vi "Activate Menu.vi"(8 "error in (no error)":errorcluster, 9 "Run Mode?":bool, 10 "MenuRef":refnum<k9>, 11 "2D Compass.lvclass in":refnum<class "2D Compass.lvclass">) -> (0 "error out":errorcluster, 3 "2D Compass.lvclass out":refnum<class "2D Compass.lvclass">)   [LabVIEW 2017, in "2D Compass.lvclass"]
uses:
  <vilib>/Math Plots/2D Math Plots/2D Compass/2D Compass/2D Compass.lvclass
  e:/builds/penguin/labview/branches/2017/dev/dist/vi.lib/Math Plots/2D Math Plots/2D Plot/2D Plot/2D Plot.lvclass
  <vilib>/Math Plots/2D Math Plots/2D Compass/2D Compass/2D Compass.lvclass/2D Compass.ctl
  <vilib>/Math Plots/2D Math Plots/2D Plot/2D Plot/2D Plot.lvclass
panel:
  in  "New Item Names":string="Auto Size Plot Legend"
  in  "Run-time Menu":T1(array[cluster])=[{"menu tag"="", "items to delete"=["APP_SC_CLEAR_GRAPH", "APP_SC_AUTOSCALE_X", "APP_SC_AUTOSCALE_Y", "APP_SC_SMOOTH_UPDATES", "APP_SC_OPTIONAL_PLANE", "APP_SC_SHOW_DIAGRAM"], "new menu"=[{"item names"="Clear Graph", "item tags"="USER_SC_CLEAR_GRAPH", "after item"="APP_SC_CLEAR_GRAPH"}, {"item names"="Autoscale Magnitude", "item tags"="USER_SC_AUTOSCALE", "after item"="APP_SEPERATOR"}], "root?"=TRUE}, {"menu tag"="APP_SC_VISIBLE_ITEMS", "items to delete"=["APP_SC_PLOT_LEGEND", "APP_SC_SCALE_LEGEND", "APP_SC_GRAPH_PALETTE", "APP_SC_CURSOR_LEGEND", "APP_SC_X_SCROLLBAR", "APP_SC_X_SCALE", "APP_SC_Y_SCALE", "APP_SC_UNIT_LABEL"], "new menu"=[{"item names"="Plot Legend", "item tags"="USER_SC_PLOT_LEGEND", "after item"="APP_SC_SEPERATOR"}, {"item names"="Scale Legend", "item tags"="USER_SC_SCALE_LEGEND", "after item"="USER_SC_PLOT_LEGEND"}, {"item names"="Graph Palette", "item tags"="USER_SC_GRAPH_PALETTE", "after item"="USER_SC_SCALE_LEGEND"}, {"item names"="Cursor Legend", "item tags"="USER_SC_CURSOR_LEGEND", "after item"="USER_SC_GRAPH_PALETTE"}, {"item names"="X Scrollbar", "item tags"="USER_SC_X_SCROLLBAR", "after item"="USER_SC_CURSOR_LEGEND"}, {"item names"="-", "item tags"="APP_SC_SEPERATOR", "after item"="USER_SC_X_SCROLLBAR"}, {"item names"="Magnitude Scale", "item tags"="USER_SC_MAGNITUDE_SCALE", "after item"="APP_SC_SEPERATOR"}, {"item names"="Phase Scale", "item tags"="USER_SC_PHASE_SCALE", "after item"="USER_SC_MAGNITUDE_SCALE"}], "root?"=FALSE}]
  in  "Edit-time Menu":T1(array[cluster])=[{"menu tag"="", "items to delete"=["APP_SC_AUTOSCALE_X", "APP_SC_AUTOSCALE_Y", "APP_SC_SMOOTH_UPDATES", "APP_SC_OPTIONAL_PLANE", "APP_SC_PROPERTIES"], "new menu"=[{"item names"="Autoscale Magnitude", "item tags"="USER_SC_AUTOSCALE", "after item"="APP_SC_AUTOSCALE_X"}, {"item names"="Properties", "item tags"="USER_SC_PROPERTIES", "after item"="APP_SC_SEPARATOR"}], "root?"=TRUE}, {"menu tag"="APP_SC_VISIBLE_ITEMS", "items to delete"=["APP_SC_PLOT_LEGEND", "APP_SC_SCALE_LEGEND", "APP_SC_GRAPH_PALETTE", "APP_SC_CURSOR_LEGEND", "APP_SC_X_SCROLLBAR", "APP_SC_X_SCALE", "APP_SC_Y_SCALE", "APP_SC_UNIT_LABEL"], "new menu"=[{"item names"="Plot Legend", "item tags"="USER_SC_PLOT_LEGEND", "after item"="APP_SC_SEPERATOR"}, {"item names"="Scale Legend", "item tags"="USER_SC_SCALE_LEGEND", "after item"="USER_SC_PLOT_LEGEND"}, {"item names"="Graph Palette", "item tags"="USER_SC_GRAPH_PALETTE", "after item"="USER_SC_SCALE_LEGEND"}, {"item names"="Cursor Legend", "item tags"="USER_SC_CURSOR_LEGEND", "after item"="USER_SC_GRAPH_PALETTE"}, {"item names"="X Scrollbar", "item tags"="USER_SC_X_SCROLLBAR", "after item"="USER_SC_CURSOR_LEGEND"}, {"item names"="-", "item tags"="APP_SC_SEPERATOR", "after item"="USER_SC_X_SCROLLBAR"}, {"item names"="Magnitude Scale", "item tags"="USER_SC_MAGNITUDE_SCALE", "after item"="APP_SC_SEPERATOR"}, {"item names"="Phase Scale", "item tags"="USER_SC_PHASE_SCALE", "after item"="USER_SC_MAGNITUDE_SCALE"}], "root?"=FALSE}, {"menu tag"="APP_SC_ADVANCED", "items to delete"=["APP_SC_SHOW_DIAGRAM"], "new menu"=[], "root?"=FALSE}]
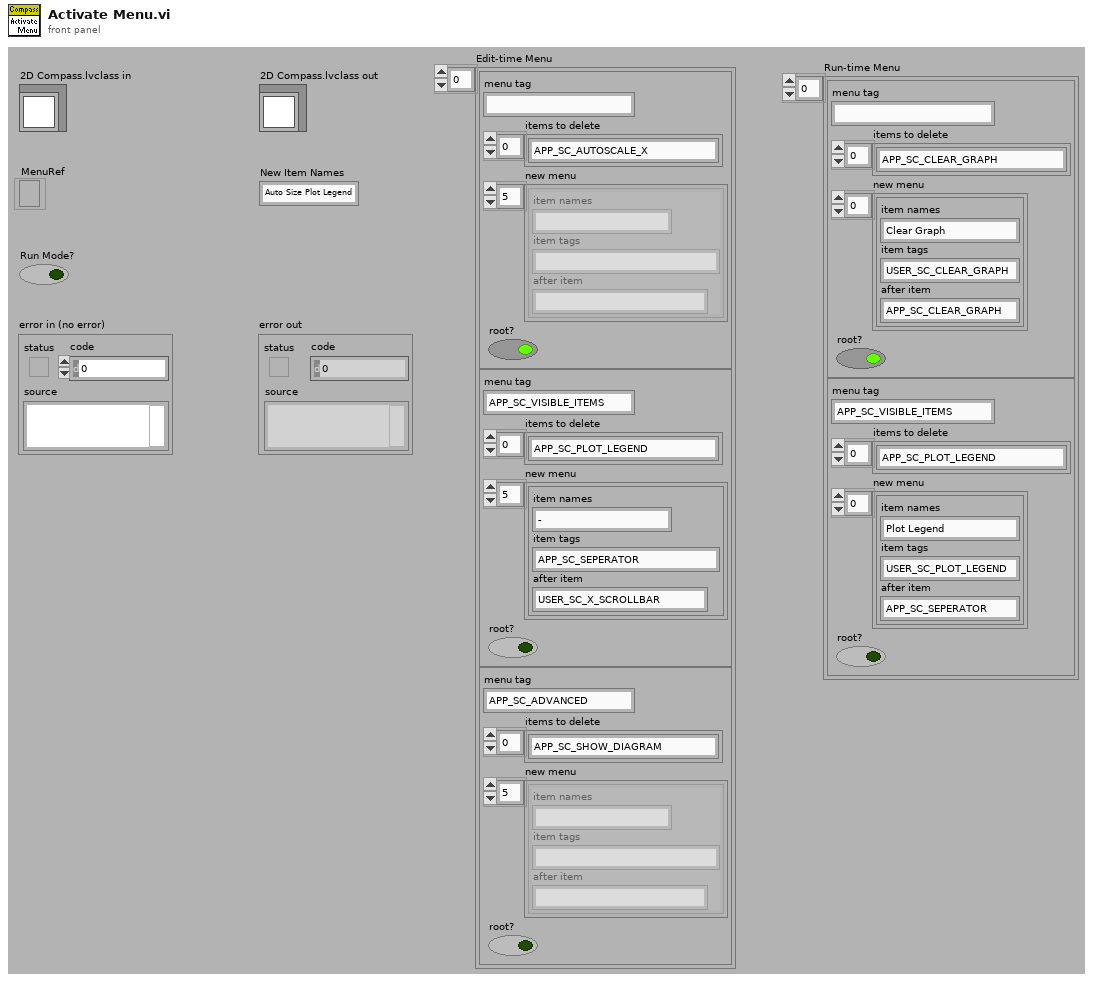
[diagram p1: front panel]
types:
  T1 = cluster{"menu tag":string, "items to delete":string[], "new menu":cluster{"item names":string, "item tags":string, "after item":string}[], "root?":bool}[]
  T2 = typedef "2D Plot.lvclass/Property Cluster.ctl" = cluster{"Graph General":T3, "Format Property":string[], "Scale Array":T4, "Cursor Property":T7, "Annotation List":T9, "Active Cursor":i32, "Active Plot":i32}
  T3 = typedef "2D Plot.lvclass/Graph General Property.ctl" = cluster{"Palette Visible":cluster{"Graph Legend":bool, "Plot Legend":bool, "Auto size":bool, "Number of Plots":u32, "X Scrollbar":bool, "Scale Legend":bool, "Cursor Legend":bool}, "Plot Area Color":cluster{"FG Color":u32, "BG Color":u32}, "Bounds Size":cluster{"Width":u32, "Height":u32}, "Plot Area Bounds":cluster{"Left":i16, "Top":i16, "Right":i16, "Bottom":i16}}
  T4 = typedef "2D Plot.lvclass/Scale Array.ctl" = T5[]
  T5 = typedef "2D Plot.lvclass/Scale Cluster.ctl" = cluster{"General":cluster{"Editable":bool, "Flipped":bool, "Mapping Mode":u8, "Visible":bool, "Style":u8, "Scale Fit":u8}, "Offset and Multiplier":T6, "Range":cluster{"Minimum":dbl, "Maximum":dbl, "Increment":dbl, "Minor Increment":dbl, "Start":dbl}, "Tick Color":cluster{"Major Color":u32, "Minor Color":u32}, "Gird Color":cluster{"Major Color":u32, "Minor Color":u32}, "Marker":cluster{"Visible":bool, "FG Color":u32, "BG Color":u32, "Font Name":string, "Font Size":u32, "Font Bold":bool, "Font Italic":bool, "Font Strikeout":bool, "Font Underline":bool}, "Name Label":cluster{"Visible":bool, "FG Color":u32, "BG Color":u32, "Font Name":string, "Font Size":u32, "Font Bold":bool, "Font Italic":bool, "Font Strikeout":bool, "Font Underline":bool, "Justification":enum16{"Left", "Center", "Right"}, "Text":string}}
  T6 = typedef "LVOffsetAndMultiplierTypeDef.ctl" = cluster{"Offset":dbl, "Multiplier":dbl}
  T7 = typedef "2D Plot.lvclass/Cursor Property.ctl" = cluster{"Cursor List":T8, "Cursor List Addtional":cluster{"Cursor Selection Color":u32, "Line Style":u8, "Line Width":u8, "Visible":bool}[]}
  T8 = typedef "LVCursorListTypeDef.ctl" = cluster{"Name":string, "Color":u32, "Style":u8, "Point Style":u8, "Name Visible":bool, "Allow Drag":bool, "Cursor Mode":u32, "Plot":i32, "Index":i32, "Position":cluster{"X":dbl, "Y":dbl}, "X Scale":u32, "Y Scale":u32, "Watch Plots":i32[], "Watch All Plots":bool, "Plot Area":i32, "Label Offset":cluster{"X":dbl, "Y":dbl}}[]
  T9 = typedef "LVAnnotationListTypeDef.ctl" = cluster{"Name":string, "Color":u32, "Style":u8, "Point Style":u8, "Name Visible":bool, "Allow Drag":bool, "Annotation Mode":u32, "Plot":i32, "Index":i32, "Position":cluster{"X":dbl, "Y":dbl}, "X Scale":u32, "Y Scale":u32, "Show Arrow":bool, "Lock Name":bool, "Plot Area":i32, "Label Offset":cluster{"X":dbl, "Y":dbl}}[]
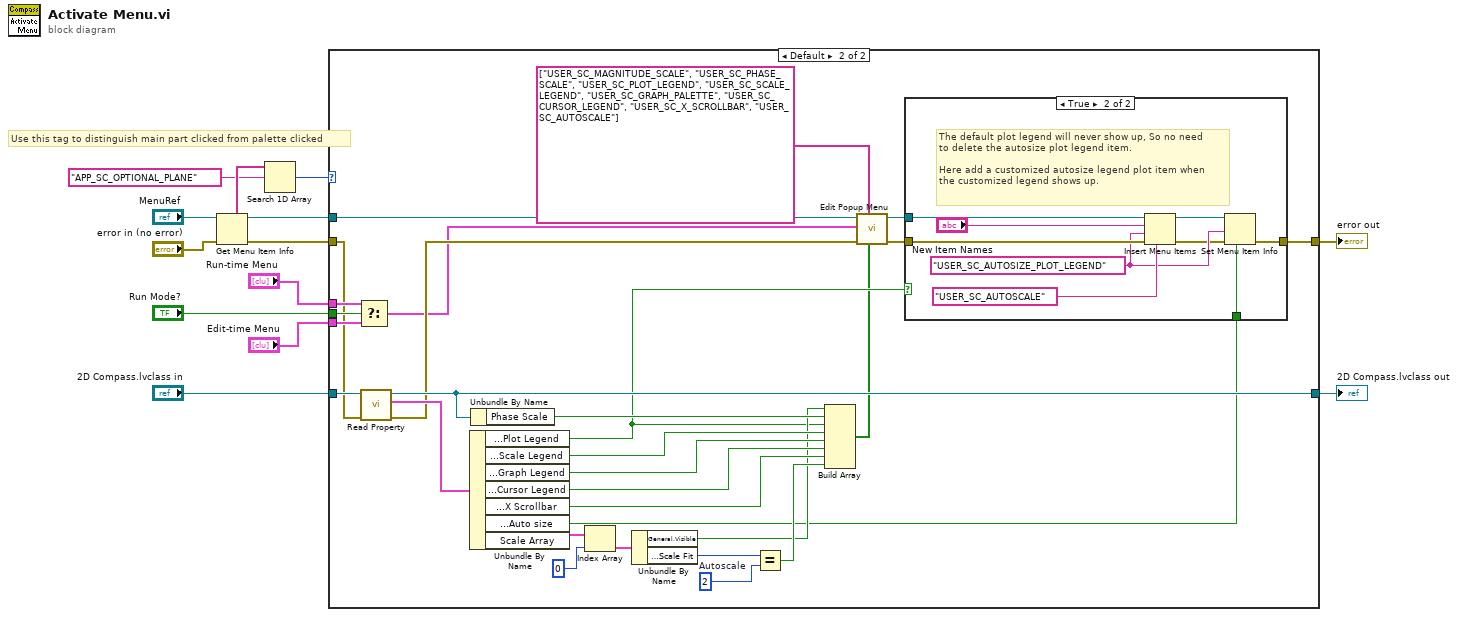
[diagram p0: block diagram]
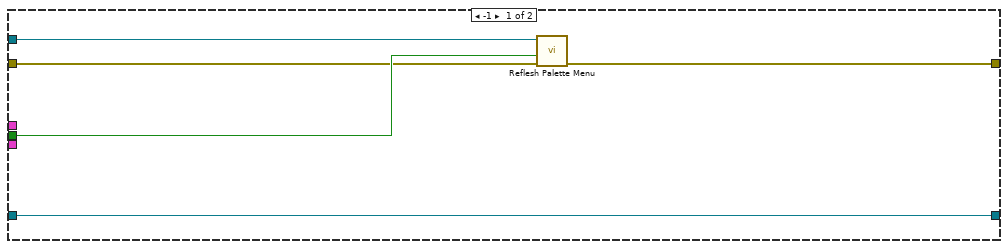
[diagram p2: hidden frame]
diagram:
  # "Use this tag to distinguish main part clicked from palette clicked"
  n1 = Get Menu Item Info(8:"error in (no error)", 11:"MenuRef") -> (0:w1:errorcluster, 3:w6:refnum<k9>, 5:w5:string[])  [unwired: 5 out]
  n2 = Search 1D Array(1D array=w5, element="APP_SC_OPTIONAL_PLANE") -> (index of element=w3:i32)  [unwired: 1 out]
  n3 = case shown="Default" w3 {
    tunnel: "2D Compass.lvclass in" -> [w18 w47]
    tunnel: "Run Mode?" -> [w16 w45]
    tunnel: "Run-time Menu" -> [_ w44]
    tunnel: "Edit-time Menu" -> [_ w43]
    tunnel: w6 -> [w17 w27]
    tunnel: w1 -> [w15 w32]
    tunnel: [w14 w31] -> w9
    tunnel: [w18 w30] -> w8
    frame -1 {
      n4 = call <vilib>:"Reflesh Palette Menu.vi"("error in (no error)"=w15, "Run Mode?"=w16, "MenuRef"=w17) -> ("error out"=w14:errorcluster)  [unwired: 8 in]
    }
    frame Default {
      w39 = u8 2  # Autoscale
      n5 = Select(t=w44, s=w45, f=w43) -> (s? t:f=w25:T1)
      n6 = call <vilib>:"Read Property.vi"("error in (no error)"=w32, "2D Plot.lvclass in"=w47) -> ("error out"=w26:errorcluster, "XY Graph Property Cluster"=w46:T2, "2D Plot.lvclass out"=w30:refnum<class "2D Compass.lvclass">)  [unwired: 7 out]
      n7 = Unbundle By Name(w46) -> ("Graph General.Palette Visible.Plot Legend"=w28:bool, "Graph General.Palette Visible.Scale Legend"=w37:bool, "Graph General.Palette Visible.Graph Legend"=w36:bool, "Graph General.Palette Visible.Cursor Legend"=w35:bool, "Graph General.Palette Visible.X Scrollbar"=w34:bool, "Graph General.Palette Visible.Auto size"=w20:bool, "Scale Array"=w42:T4)
      n8 = Unbundle By Name(w30) -> ("Phase Scale"=w38:bool)
      n9 = Index Array(array=w42, index=0) -> (element=w41:T5)
      n10 = Unbundle By Name(w41) -> ("General.Visible"=w29:bool, "General.Scale Fit"=w40:u8)
      n11 = Equal?(x=w40, y=w39) -> (x = y?=w33:bool)
      n12 = Build Array(w29, w38, w28, w37, w36, w35, w34, w33) -> (w23:bool[])
      n13 = call <vilib>:"Edit Popup Menu.vi"("User Menu States"=w23, "User Menu Items"=string[] ["USER_SC_MAGNITUDE_SCALE", "USER_SC_PHASE_SCALE", "USER_SC_PLOT_LEGEND", "USER_SC_SCALE_LEGEND", "USER_SC_GRAPH_PALETTE", "USER_SC_CURSOR_LEGEND", "USER_SC_X_SCROLLBAR", "USER_SC_AUTOSCALE"] ("Array"), "error in (no error)"=w26, "Menu Operation Cluster"=w25, "Menu Ref In"=w27) -> ("error out"=w21:errorcluster, "Menu Ref Out"=w22:refnum<k9>)  [unwired: 5 out]
      n14 = case shown="True" w28 {
        tunnel: w22 -> [_ w57]
        tunnel: w21 -> [w48 w54]
        tunnel: [w48 w49] -> w31
        tunnel: w20 -> [_ w51]
        frame False {
        }
        frame True {
          w52 = "USER_SC_AUTOSIZE_PLOT_LEGEND"
          # "The default plot legend will never show up, So no need\nto delete the autosize plot legend item.\n\nHere add a customized autosize legend plot item when\nthe customized legend shows up."
          n15 = Insert Menu Items(4:"USER_SC_AUTOSCALE" ("after item"), 6:w54, 7:w52, 8:"New Item Names", 9:w57) -> (0:w50:errorcluster, 3:w53:refnum<k9>)  [unwired: 2 out]
          n16 = Set Menu Item Info(6:w51, 7:w52, 8:w50, 11:w53) -> (0:w49:errorcluster)  [unwired: 4 out]
        }
      }
    }
  }
  "error out" <- w9
  "2D Compass.lvclass out" <- w8
